vi "counter_and_averaging_sr_examples.vi"() -> ()   [LabVIEW 2023]
panel:
  out "Waveform Graph":dbl[][](graph)
  in  "Stop Button":bool
  out "Counter":i32
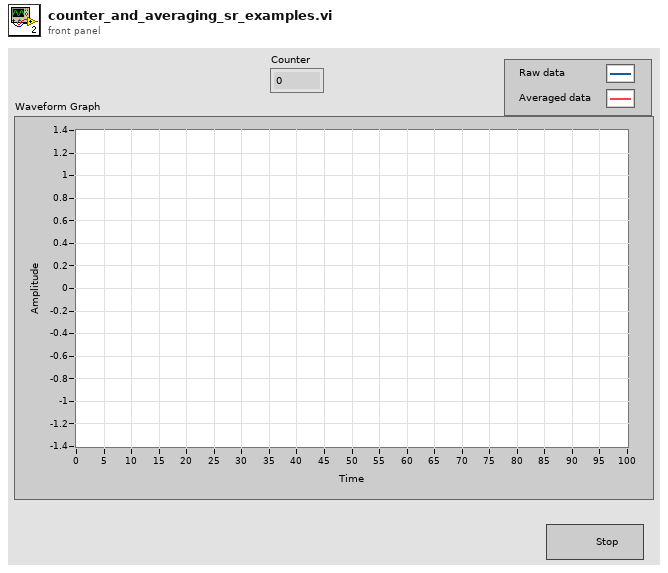
[diagram p1: front panel]
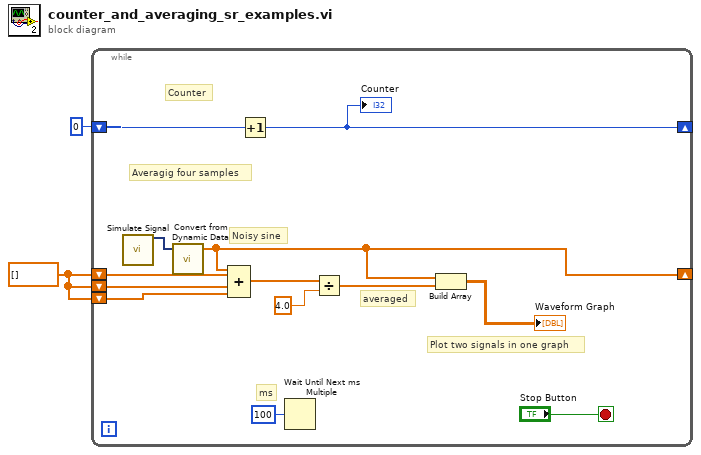
[diagram p0: block diagram]
diagram:
  w1 = dbl[] []
  n1 = while {
    shift-right: [w14] -> _
    shift-left: 0 -> [w15]
    shift-right: [w4] -> _
    shift-left: w1 -> [w12]
    shift-left: w1 -> [w11]
    shift-left: w1 -> [w10]
    stop <- "Stop Button" stop-if-true
    # "Plot two signals in one graph"
    # "averaged"
    # "Noisy sine"
    # "ms"
    # "Averagig four samples"
    # "Counter"
    n2 = call "Simulate Signal"() -> ("Sine with Uniform Noise"=w5:dynamicdata)  [unwired: 14 in, 1 out]
    n3 = call "Convert from Dynamic Data"("Dynamic Data Type"=w5) -> ("Array"=w4:dbl[])  [unwired: 3 in]
    n4 = Compound Arithmetic op=ADD(w4, w12, w11, w10) -> (w9:dbl[])
    n5 = Increment(x=w15) -> (x+1=w14:i32)
    "Counter" <- w14
    n6 = Wait Until Next ms Multiple(millisecond multiple=u32 100) -> ()  [unwired: 1 out]
    n7 = Divide(x=w9, y=4.0) -> (x/y=w7:dbl[])
    n8 = Build Array "Build Array"(w4, w7) -> (→"Waveform Graph":dbl[][])
  }
